vi "FTW-JSON-Object-Keys.vi"(0 "JSON Object":refnum<data-value>, 11 "error in":errorcluster) -> (4 "JSON Object out":refnum<data-value>, 6 "Keys":string[](array[string]), 15 "error out":errorcluster)   [LabVIEW 2015]
uses:
  core/FTW-JSON-Core-Structure.ctl
panel:
  # "Inputs"
  # "Outputs"
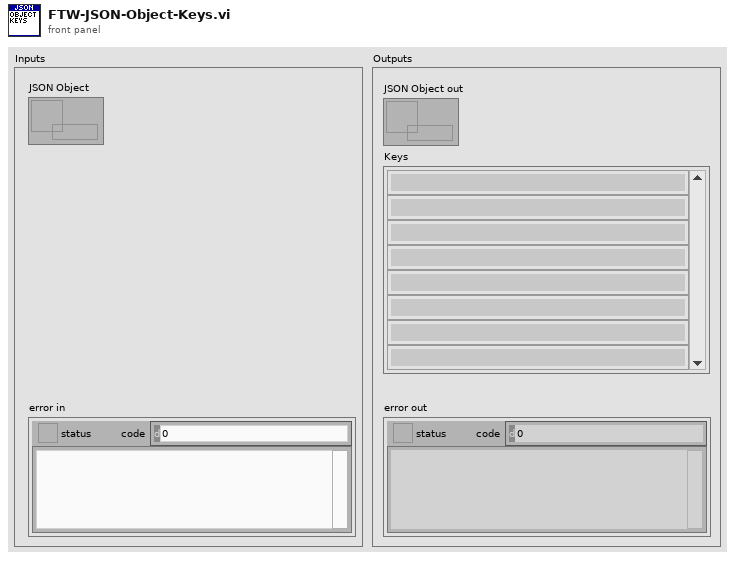
[diagram p1: front panel]
types:
  T1 = typedef "FTW-JSON-Core-Structure.ctl" = cluster{"JSON Object":i64, "Encoding Flags":i64, "Decoding Flags":i64}
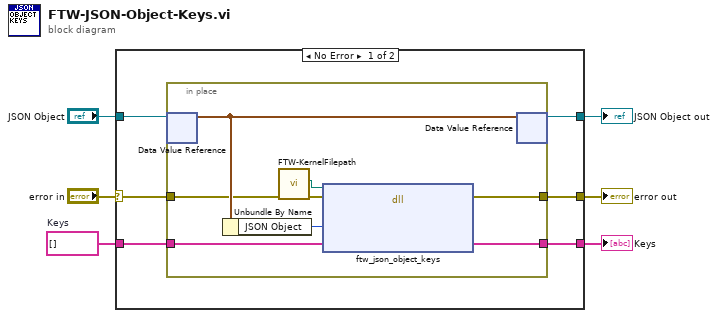
[diagram p0: block diagram]
diagram:
  w1 = string[] []  # Keys
  n1 = case shown="No Error" "error in" {
    selector: "error in" -> [w10 w22]
    tunnel: [w12 w22] -> w6
    tunnel: [w8 w21] -> w4
    tunnel: "JSON Object" -> [w9 w21]
    tunnel: [w11 _] -> w2
    tunnel: w1 -> [w7 _]
    frame No Error {
      n2 = in-place {
        in-place-border: [w16] -> w12
        in-place-border: [w17] -> w11
        in-place-border: w10 -> [w15]
        in-place-border: w7 -> [w18]
        n3 = in-place-dvr #1(w9) -> (w19:T1)  [unwired: 1 out]
        n4 = Unbundle By Name(w19) -> ("JSON Object"=w20:i64)
        n5 = call "FTW-KernelFilepath.vi"("error in"=w15) -> ("error out"=w14:errorcluster, "Library Filepath"=w13:path)  [unwired: 8 in, 1 out]
        n6 = dll-call lib="?" fn="ftw_json_object_keys"(path in=w13, error in=w14, "JSON Object Pointer"=w20, "Keys"=w18) -> (error out=w16:errorcluster, "Keys"=w17:string[])  [unwired: 3 in, 1 out]
        n7 = in-place-dvr #1(w19) -> (w8:refnum<data-value>)  [unwired: 1 out]
      }
    }
    frame Error {
    }
  }
  "error out" <- w6
  "JSON Object out" <- w4
  "Keys" <- w2
